vi "信息框（标题、文本、图标）.vi"(7 "icon":i32(ring) items=["None"=0, "Hand, Error, Stop"=16, "Question"=32, "Exclamation, Warning"=48, "Asterisk, Information"=64], 8 "错误输入（无错误）":errorcluster, 9 "buttons":i32(ring) items=["OK", "OKCancel", "AbortRetryIgnore", "YesNoCancel", "YesNo", "RetryCancel"], 10 "caption":string, 11 "text":string) -> (0 "错误输出":errorcluster, 3 "按钮输出":i32(ring) items=["None", "OK", "Cancel", "Abort", "Retry", "Ignore", "Yes", "No"])   [LabVIEW 2020]
uses:
  System.Windows.Forms
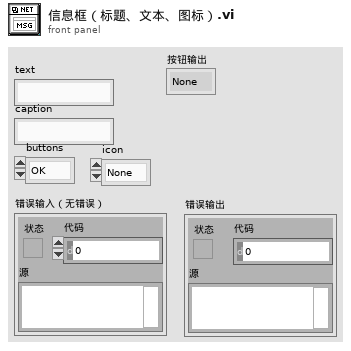
[diagram p1: front panel]
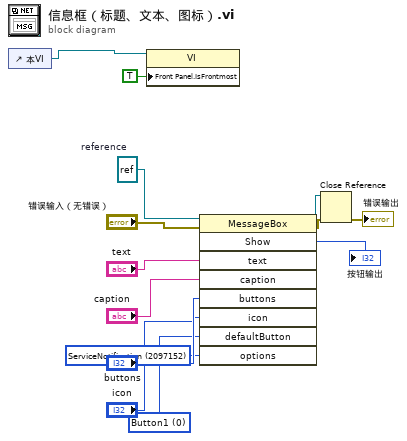
[diagram p0: block diagram]
diagram:
  w1 = 2097152 items=["DefaultDesktopOnly"=131072, "RightAlign"=524288, "RtlReading"=1048576, "ServiceNotification"=2097152] ("options")
  w2 = 0 items=["Button1"=0, "Button2"=256, "Button3"=512] ("defaultButton")
  w10 = refnum<k24> refnum  # reference
  n1 = control-ref of="本VI"() -> (w6:refnum<vi>)
  n2 = property class="VI"(reference=w6, "Front Panel.IsFrontmost"=TRUE ("前面板窗口:在最前")) -> ()  [unwired: 1 in, 2 out]
  n3 = invoke class="MessageBox" method="Show"(reference=w10, error in="错误输入（无错误）", "text"="text", "caption"="caption", "buttons"="buttons", "icon"="icon", "defaultButton"=w2, "options"=w1) -> (reference out=w14:refnum<k24>, error out=w13:errorcluster, "Show"=→"按钮输出":i32)  [unwired: 1 in, 6 out]
  n4 = Close Reference(reference=w14, error in (no error)=w13) -> (error out=→"错误输出":errorcluster)
